vi "TransmitString.vi"(8 "error in (no error)":errorcluster, 10 "string to transmit":string, 11 "queue cluster":T1) -> (0 "error out":errorcluster, 3 "queue cluster out":T1)   [LabVIEW 2014]
uses:
  typedefs/clientStatus.ctl
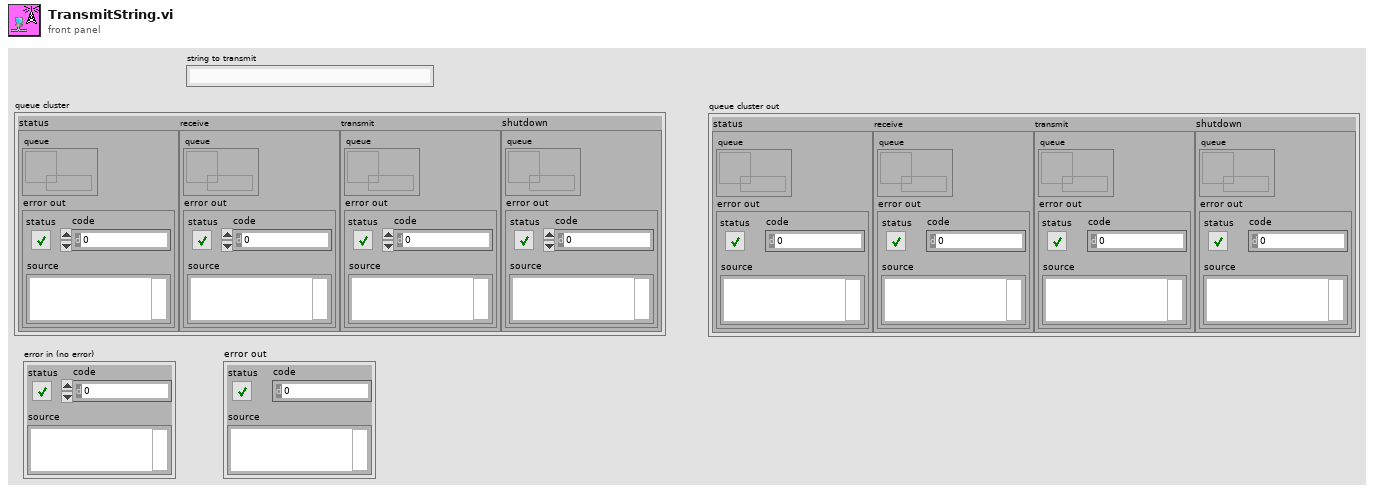
[diagram p1: front panel]
types:
  T1 = cluster{"status":cluster{"queue":refnum<queue>, "error out":errorcluster}, "receive":cluster{"queue":refnum<queue>, "error out":errorcluster}, "transmit":cluster{"queue":refnum<queue>, "error out":errorcluster}, "shutdown":cluster{"queue":refnum<queue>, "error out":errorcluster}}
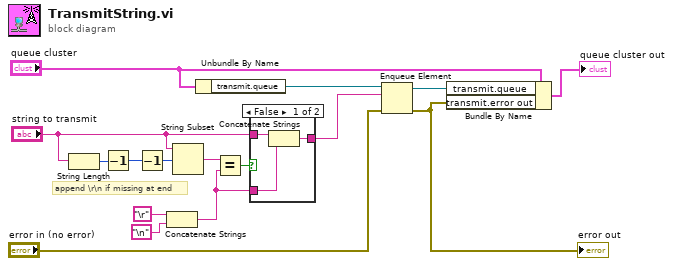
[diagram p0: block diagram]
diagram:
  # "append \\r\\n if missing at end"
  n1 = String Length(string="string to transmit") -> (length=w10:i32)
  n2 = Decrement(x=w10) -> (x-1=w9:i32)
  n3 = Decrement(x=w9) -> (x-1=w3:i32)
  n4 = Concatenate Strings("\r", "\n") -> (w2:string)
  n5 = String Subset(string="string to transmit", offset (0)=w3) -> (substring=w8:string)  [unwired: 1 in]
  n6 = Unbundle By Name("queue cluster") -> ("transmit.queue"=w16:refnum<queue>)
  n7 = Equal?(x=w8, y=w2) -> (x = y?=w7:bool)
  n8 = case shown="False" w7 {
    tunnel: "string to transmit" -> [w18 w20]
    tunnel: [w19 w20] -> w5
    tunnel: w2 -> [w17 _]
    frame False {
      n9 = Concatenate Strings(w18, w17) -> (w19:string)
    }
    frame True {
    }
  }
  n10 = Enqueue Element(queue=w16, element=w5, error in (no error)="error in (no error)") -> (queue out=w11:refnum<queue>, error out=w12:errorcluster)  [unwired: 1 in, 1 out]
  "error out" <- w12
  n11 = Bundle By Name(cluster="queue cluster", "transmit.queue"=w11, "transmit.error out"=w12) -> (→"queue cluster out":T1)
